vi "calculate path.vi"() -> (3 "Path":path=path "C:/Users/Daniel/Source/Repos/paho.mqtt.c/LVMQTT/paho-mqtt3a.*")   [LabVIEW 2014, in "MQTT client.lvclass"]
uses:
  MQTT client.lvclass
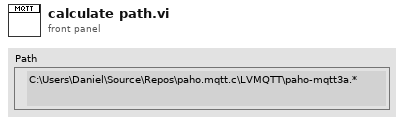
[diagram p1: front panel]
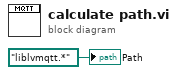
[diagram p0: block diagram]
diagram:
  "Path" <- path "liblvmqtt.*"
